vi "Tutorial 03.vi"() -> ()   [LabVIEW 2014]
panel:
  out "f(x)":dbl
  in  "x":dbl
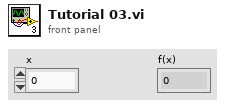
[diagram p1: front panel]
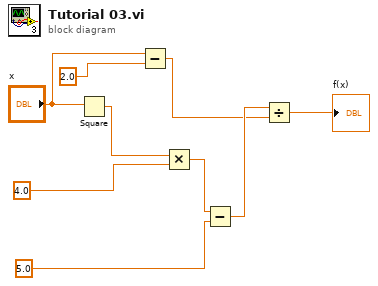
[diagram p0: block diagram]
diagram:
  n1 = Square(x="x") -> (x^2=w9:dbl)
  n2 = Subtract(x="x", y=2.0) -> (x-y=w2:dbl)
  n3 = Multiply(x=w9, y=4.0) -> (x*y=w7:dbl)
  n4 = Subtract(x=w7, y=5.0) -> (x-y=w3:dbl)
  n5 = Divide(x=w3, y=w2) -> (x/y=→"f(x)":dbl)
